vi "CheckServers.vi"(10 "kill":bool) -> ()   [LabVIEW 2013]
uses:
  _ROSDefinition.vi
panel:
  out "error out":errorcluster
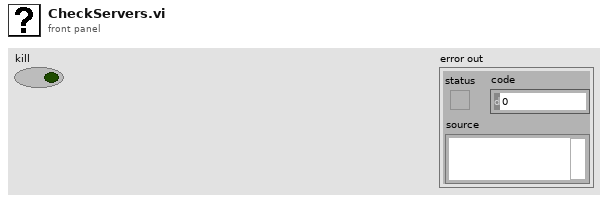
[diagram p1: front panel]
types:
  T1 = cluster{"server vi":string, "reference":refnum<vi>, "Description":string[], "Connected":bool}[]
  T2 = enum32{"Bad", "Idle", "Run top level", "Running"}
  T3 = cluster{"server vi":string, "reference":refnum<vi>, "Description":string[], "Connected":bool}
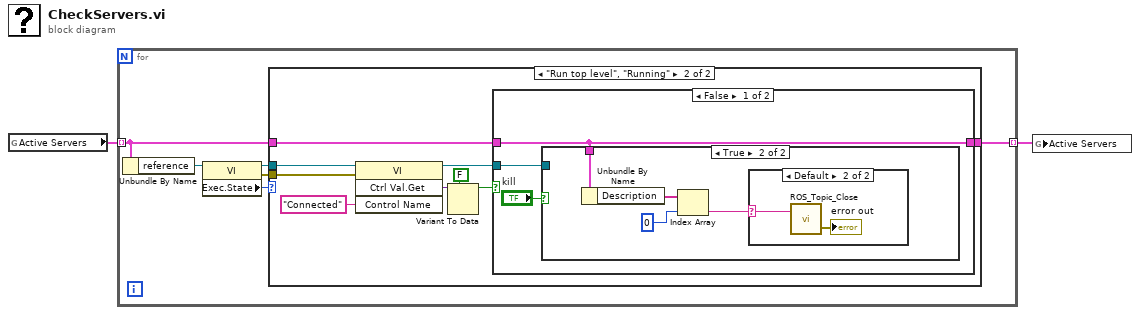
[diagram p0: block diagram]
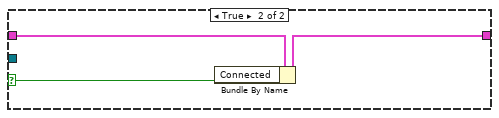
[diagram p5: hidden frame]
diagram:
  n1 = global read "_ROSDefinition.vi" "Active Servers"() -> (w2:T1)
  n2 = for {
    tunnel: w2 -> [w6] mode=indexing
    tunnel: [w3] -> w1 mode=indexing
    n3 = Unbundle By Name(w6) -> ("reference"=w8:refnum<vi>)
    n4 = property class="VI"(reference=w8) -> (reference out=w5:refnum<vi>, error out=w4:errorcluster, "Exec.State"=w7:T2)  [unwired: 1 in]
    n5 = case shown="\"Run top level\", \"Running\"" w7 {
      tunnel: w6 -> [w9 w14]
      tunnel: w5 -> [_ w18]
      tunnel: w4 -> [_ w17]
      tunnel: [w9 w13] -> w3
      frame "Bad", Default {
      }
      frame "Run top level", "Running" {
        n6 = invoke class="VI" method="Ctrl Val.Get"(reference=w18, error in=w17, "Control Name"="Connected") -> (reference out=w12:refnum<vi>, "Get Control Value Variant"=w15:variant)  [unwired: 1 in, 2 out]
        n7 = Variant To Data(type=FALSE, Variant=w15) -> (data=w10:bool)  [unwired: 1 in, 1 out]
        n8 = case shown="False" w10 {
          selector: w10 -> [_ w28]
          tunnel: w14 -> [w19 w30]
          tunnel: [w19 w29] -> w13
          tunnel: w12 -> [w21 _]
          frame False {
            n9 = case shown="True" "kill" {
              tunnel: w21 -> [_ _]
              tunnel: w19 -> [_ w23]
              frame False {
              }
              frame True {
                n10 = Unbundle By Name(w23) -> ("Description"=w25:string[])
                n11 = Index Array(array=w25, index=0) -> (element=w22:string)
                n12 = case shown="Default" w22 {
                  selector: w22 -> [_ w26]
                  frame "/labview" {
                    # "don't kill /labview"
                  }
                  frame Default {
                    n13 = call "ROS_Topic_Close.vi"("topic"=w26) -> ("error out"=→"error out":errorcluster)  [unwired: 3 in]
                  }
                }
              }
            }
          }
          frame True {
            n14 = Bundle By Name(cluster=w30, "Connected"=w28) -> (w29:T3)
          }
        }
      }
    }
  }
  n15 = global write "_ROSDefinition.vi" "Active Servers"(w1) -> ()
